vi "Get BC Array Size.vi"(8 "error in (no error)":errorcluster, 11 "PDE_Heat_2D in":refnum<class "NI_PDE_Heat_2D.lvclass">) -> (0 "error out":errorcluster, 2 "# of BC":i32, 3 "PDE_Heat_2D out":refnum<class "NI_PDE_Heat_2D.lvclass">)   [LabVIEW 2020, in "NI_PDE.lvlib" / "NI_PDE_Heat_2D.lvclass"]
uses:
  <vilib>/gmath/pde.llb/PDEClass/PDE_Heat_2D/NI_PDE_Heat_2D.lvclass
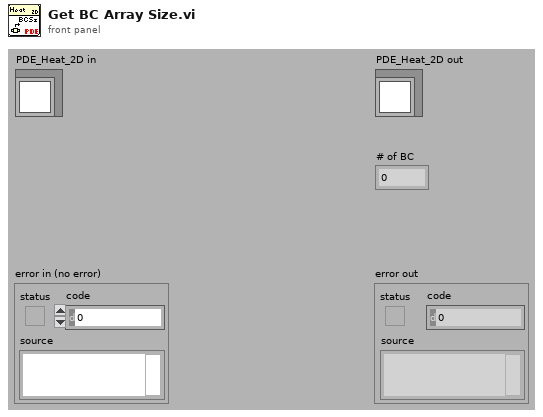
[diagram p1: front panel]
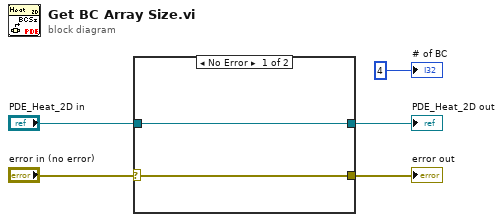
[diagram p0: block diagram]
diagram:
  n1 = case shown="No Error" "error in (no error)" {
    selector: "error in (no error)" -> [w6 w9]
    tunnel: "PDE_Heat_2D in" -> [w7 w8]
    tunnel: [w7 w8] -> w4
    tunnel: [w6 w9] -> w3
    frame No Error {
    }
    frame Error {
    }
  }
  "PDE_Heat_2D out" <- w4
  "error out" <- w3
  "# of BC" <- 4 ("# of BC")
